vi "Adiciona_valor_inicial.vi"(1 "Array":dbl[][](array[numeric]), 2 "system model in":T1 {"grey trans func spec"."# of zeros/poles at origin"."zeros/poles" items=["zeros", "poles"]; "std of zeros-poles (noise)"."gain" format="%.2f"; "std of zeros-poles (noise)"."poles" format="%.2f"; "std of zeros-poles (noise)"."zeros" format="%.2f"; "zeros-poles (noise)"."gain" format="%.2f"; "zeros-poles (noise)"."poles" format="%.2f"; "zeros-poles (noise)"."zeros" format="%.2f"; "std of trans func (noise)"."alphas" format="%.2f"; "std of trans func (noise)"."betas" format="%.2f"; "trans func (noise)"."alphas" format="%.2f"; "trans func (noise)"."betas" format="%.2f"; "std of zeros-poles"."gain" format="%.2f"; "std of zeros-poles"."poles" format="%.2f"; "std of zeros-poles"."zeros" format="%.2f"; "std of trans func"."alphas" format="%.2f"; "std of trans func"."betas" format="%.2f"; "zeros-poles"."gain" format="%.2f"; "zeros-poles"."poles" format="%.2f"; "zeros-poles"."zeros" format="%.2f"; "trans func"."alphas" format="%.2f"; "trans func"."betas" format="%.2f"; "fs" format="%.2f"; "std deviations"."A" format="%.2f"; "std deviations"."D" format="%.2f"; "std deviations"."C" format="%.2f"; "std deviations"."F" format="%.2f"; "std deviations"."B" format="%.2f"; "coefficients"."A" format="%.2f"; "coefficients"."D" format="%.2f"; "coefficients"."C" format="%.2f"; "coefficients"."F" format="%.2f"; "coefficients"."B" format="%.2f"; "attributes"."model type" items=["Undefined", "AR", "ARX (SISO)", "ARX (MISO)", "ARX (MIMO)", "ARMAX (SISO)", "ARMAX (MISO)", "Output-Error (SISO)", "Output-Error (MISO)", "Box-Jenkins (SISO)", "Box-Jenkins (MISO)", "General Linear (SISO)", "General Linear (MISO)", "State-Space (SISO)", "State-Space (MISO)", "State-Space (MIMO)", "Transfer Function (SISO)", "Transfer Function (MISO)", "Transfer Function (MIMO)", "Zero-Pole-Gain (SISO)", "Zero-Pole-Gain (MISO)", "Zero-Pole-Gain (MIMO)"]}) -> (0 "system model out":T1 {"grey trans func spec"."# of zeros/poles at origin"."zeros/poles" items=["zeros", "poles"]; "std of zeros-poles (noise)"."gain" format="%.2f"; "std of zeros-poles (noise)"."poles" format="%.2f"; "std of zeros-poles (noise)"."zeros" format="%.2f"; "zeros-poles (noise)"."gain" format="%.2f"; "zeros-poles (noise)"."poles" format="%.2f"; "zeros-poles (noise)"."zeros" format="%.2f"; "std of trans func (noise)"."alphas" format="%.2f"; "std of trans func (noise)"."betas" format="%.2f"; "trans func (noise)"."alphas" format="%.2f"; "trans func (noise)"."betas" format="%.2f"; "std of zeros-poles"."gain" format="%.2f"; "std of zeros-poles"."poles" format="%.2f"; "std of zeros-poles"."zeros" format="%.2f"; "std of trans func"."alphas" format="%.2f"; "std of trans func"."betas" format="%.2f"; "zeros-poles"."gain" format="%.2f"; "zeros-poles"."poles" format="%.2f"; "zeros-poles"."zeros" format="%.2f"; "trans func"."alphas" format="%.2f"; "trans func"."betas" format="%.2f"; "fs" format="%.2f"; "std deviations"."A" format="%.2f"; "std deviations"."D" format="%.2f"; "std deviations"."C" format="%.2f"; "std deviations"."F" format="%.2f"; "std deviations"."B" format="%.2f"; "coefficients"."A" format="%.2f"; "coefficients"."D" format="%.2f"; "coefficients"."C" format="%.2f"; "coefficients"."F" format="%.2f"; "coefficients"."B" format="%.2f"; "attributes"."model type" items=["Undefined", "AR", "ARX (SISO)", "ARX (MISO)", "ARX (MIMO)", "ARMAX (SISO)", "ARMAX (MISO)", "Output-Error (SISO)", "Output-Error (MISO)", "Box-Jenkins (SISO)", "Box-Jenkins (MISO)", "General Linear (SISO)", "General Linear (MISO)", "State-Space (SISO)", "State-Space (MISO)", "State-Space (MIMO)", "Transfer Function (SISO)", "Transfer Function (MISO)", "Transfer Function (MIMO)", "Zero-Pole-Gain (SISO)", "Zero-Pole-Gain (MISO)", "Zero-Pole-Gain (MIMO)"]})   [LabVIEW 2018]
uses:
  <vilib>/addons/System Identification/Model Typedefs.llb/si_generic model.ctl
  <vilib>/addons/System Identification/Model Typedefs.llb/SI Model Type.ctl
  <vilib>/addons/System Identification/Model Typedefs.llb/si_variables.ctl
  <vilib>/addons/System Identification/NI_SysID.lvlib
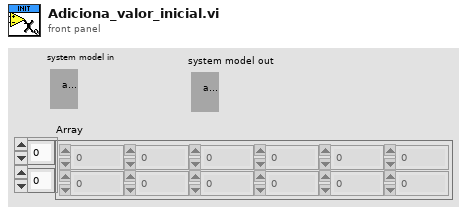
[diagram p1: front panel]
types:
  T1 = typedef "NI_SysID.lvlib/si_generic model.ctl" = cluster{"attributes":cluster{"version":string, "model type":T2, "input names":string[], "output names":string[], "notes":string}, "coefficients":cluster{"A ":dbl[][][], "B":dbl[][][], "F":dbl[][][], "C":dbl[][][], "D":dbl[][][]}, "std deviations":cluster{"A ":dbl[][][], "B":dbl[][][], "F":dbl[][][], "C":dbl[][][], "D":dbl[][][]}, "coefficients covariance":dbl[][][], "noise variance":dbl[][], "fs":dbl, "system info":cluster{"number of inputs":i32, "number of outputs":i32, "A order":i32[][], "B order":i32[][], "F order":i32[][], "C order":i32[][], "D order":i32[][], "Delays":i32[][]}, "kalman gain":dbl[][], "initial state":dbl[], "trans func":cluster{"betas":dbl[], "alphas":dbl[]}[][], "zeros-poles":cluster{"zeros":cdb[], "poles":cdb[], "gain":dbl}[][], "std of trans func":cluster{"betas":dbl[], "alphas":dbl[]}[][], "std of zeros-poles":cluster{"zeros":cdb[], "poles":cdb[], "gain":dbl}[][], "trans func (noise)":cluster{"betas":dbl[], "alphas":dbl[]}[][], "std of trans func (noise)":cluster{"betas":dbl[], "alphas":dbl[]}[][], "zeros-poles (noise)":cluster{"zeros":cdb[], "poles":cdb[], "gain":dbl}[][], "std of zeros-poles (noise)":cluster{"zeros":cdb[], "poles":cdb[], "gain":dbl}[][], "Symbolic State Space Model":cluster{"Symbolic A":string[][], "Symbolic B":string[][], "Symbolic C":string[][], "Symbolic D":string[][], "Symbolic K":string[][], "Symbolic Initial State":string[]}, "delay":dbl[][], "variables":T3, "grey trans func spec":cluster{"orders of TF model":cluster{" num order":i32, "den order":i32}, "# of zeros/poles at origin":cluster{"zeros/poles":u16, "number ":i32}, "delay initial?":bool, "gain initial?":bool}}
  T2 = typedef "NI_SysID.lvlib/SI Model Type.ctl" = u16
  T3 = typedef "NI_SysID.lvlib/si_variables.ctl" = cluster{"name":string, "initial guess":dbl, "upper limit":dbl, "lower limit":dbl, "value":dbl}[]
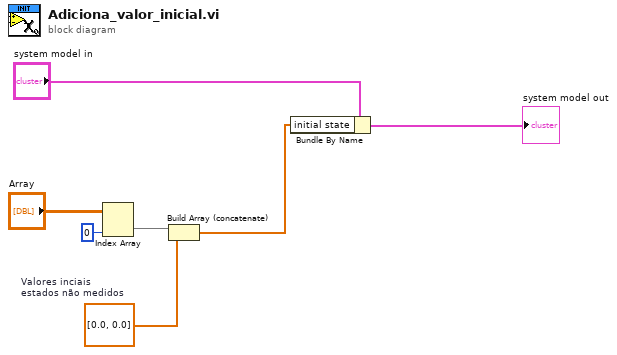
[diagram p0: block diagram]
diagram:
  w4 = dbl[] [0.0, 0.0]  # Valores inciais estados não medidos
  n1 = Index Array(array="Array", index (col)=0 ("disabled index (col)")) -> (element=w5:dbl[])  [unwired: 1 in]
  n2 = Build Array (concatenate)(w5, w4) -> (w1:dbl[])
  n3 = Bundle By Name(cluster="system model in", "initial state"=w1) -> (→"system model out":T1)
